vi "QueueCreate.vi"(8 "error in (no error)":errorcluster, 11 "Execute":refnum<class "Execute.lvclass">) -> (0 "error out":errorcluster, 3 "Execute":refnum<class "Execute.lvclass">)   [LabVIEW 2018, in "QMH_Class.lvlib" / "TestManager.lvlib" / "Execute.lvclass"]
uses:
  Execute.lvclass
  Message_class/InterfaceMessage/Interface Message.lvclass
  Execute.lvclass/Execute.ctl
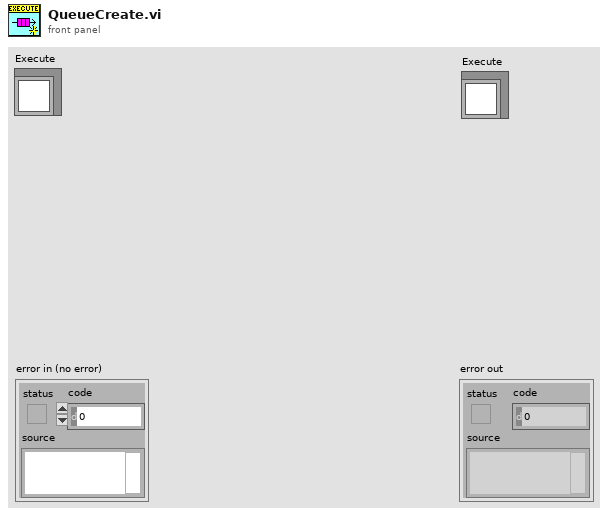
[diagram p1: front panel]
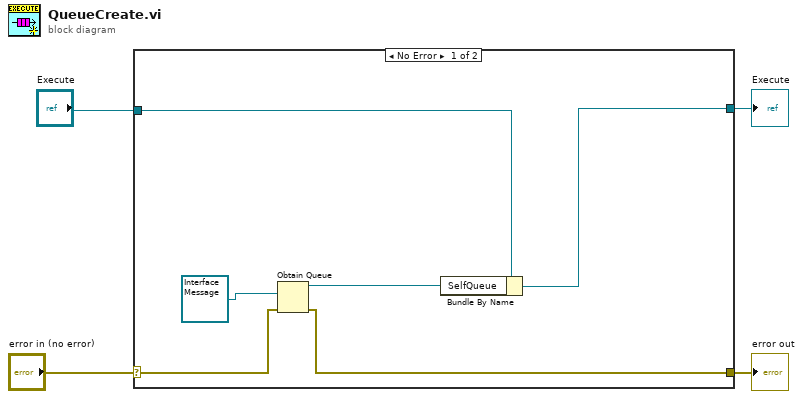
[diagram p0: block diagram]
diagram:
  n1 = case shown="No Error" "error in (no error)" {
    selector: "error in (no error)" -> [w9 w12]
    tunnel: [w8 w12] -> w3
    tunnel: [w10 w11] -> w2
    tunnel: "Execute" -> [w5 w11]
    frame No Error {
      n2 = Obtain Queue(element data type=refnum<class "Interface Message.lvclass"> refnum ("QMH_Class.lvlib:TestManager.lvlib:Interface Message.lvclass"), error in (no error)=w9) -> (queue out=w7:refnum<queue>, error out=w8:errorcluster)  [unwired: 3 in, 1 out]
      n3 = Bundle By Name(cluster=w5, "SelfQueue"=w7) -> (w10:refnum<class "Execute.lvclass">)
    }
    frame Error {
    }
  }
  "error out" <- w3
  "Execute" <- w2
